vi "get_config_cluster.vi"(8 "error in (no error)":errorcluster, 11 "ClockDL100201DAQmx in":refnum<class "ClockDL100201DAQmx.lvclass">) -> (0 "error out":errorcluster, 2 "config cluster (variant)":variant, 3 "ClockDL100201DAQmx out":refnum<class "ClockDL100201DAQmx.lvclass">)   [LabVIEW 2010, in "ClockDL100201DAQmx.lvclass"]
uses:
  ClockDL100201DAQmx.lvclass
  ClockDL100201DAQmx.lvclass/ClockDL100201DAQmx.ctl
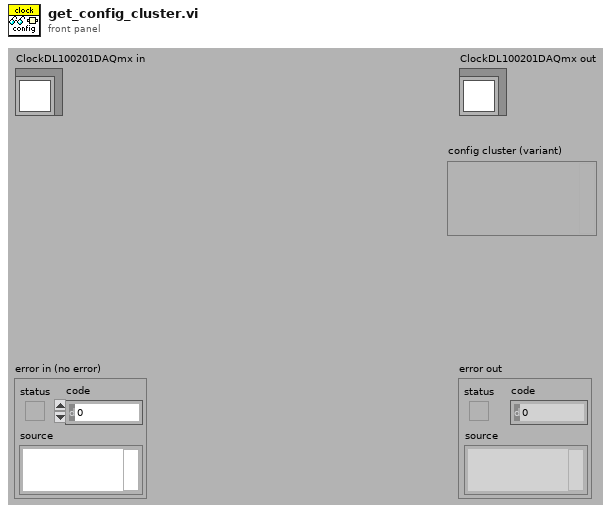
[diagram p1: front panel]
types:
  T1 = typedef "ClockDL100201DAQmx.lvclass/config_data_cluster.ctl" = cluster{"source":string, "destination":string, "counter":string}
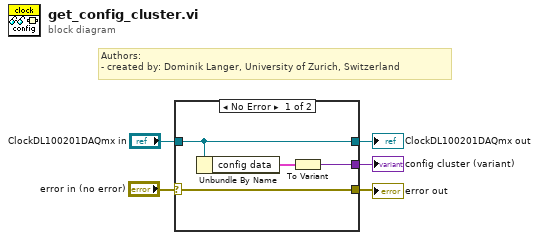
[diagram p0: block diagram]
diagram:
  # "Authors: \n- created by: Dominik Langer, University of Zurich, Switzerland"
  n1 = case shown="No Error" "error in (no error)" {
    selector: "error in (no error)" -> [w9 w11]
    tunnel: [w9 w11] -> w4
    tunnel: "ClockDL100201DAQmx in" -> [w8 w10]
    tunnel: [w8 w10] -> w2
    tunnel: [w6 _] -> w1
    frame No Error {
      n2 = Unbundle By Name(w8) -> ("config data"=w7:T1)
      n3 = To Variant(anything=w7) -> (Variant=w6:variant)
    }
    frame Error {
    }
  }
  "error out" <- w4
  "ClockDL100201DAQmx out" <- w2
  "config cluster (variant)" <- w1
